vi "Periodic Tasks.vi"(8 "error in":errorcluster) -> ()   [LabVIEW 2016]
doc: "This VI runs in parallel to other tasks. It can contain as many user-defined periodic loops as you need. These can carry out PID or other sorts of timed response."
uses:
  Common Code/Goal Vision Packet.ctl
  Common Code/Utilities/TimeManager.vi
  Common Code/Utilities/Change Detect.vi
  Common Code/Utilities/Change Detect Boolean.vi
  Robot Global Data.vi
  <vilib>/Rock Robotics/WPI/Utilities/WPI_GetSetVariantRefNum.vi
panel:
  # "e"
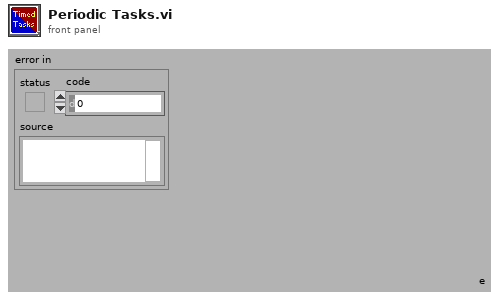
[diagram p1: front panel]
types:
  T1 = typedef "WPI_DriverStationRobotMode2.ctl" = enum16{"Autonomous Disabled", "Autonomous Enabled", "Teleop Disabled", "Teleop Enabled", "Disconnected", "Finish", "Test Disabled", "Test Enabled", "Emergency Stopped"}
  T2 = typedef "WPI_JoystickDevRef.ctl" = cluster{"Device":T3}
  T3 = typedef "WPI_JoystickDeviceEnum.ctl" = enum16{"USB 0", "USB 1", "USB 2", "USB 3", "USB 4", "USB 5"}
  T4 = typedef "D-Pad.ctl" = cluster{"Top":bool, "Bottom":bool, "None":bool, "Right":bool, "Left":bool}
  T5 = typedef "Button Cluster.ctl" = cluster{"Buttons[0]":bool, "Buttons[1]":bool, "Buttons[2]":bool, "Buttons[3]":bool, "Buttons[4]":bool, "Buttons[5]":bool, "Buttons[6]":bool, "Buttons[7]":bool, "Buttons[8]":bool, "Buttons[9]":bool}
  T6 = typedef "Goal Vision Packet.ctl" = cluster{"Distance":dbl, "Angle":dbl, "Found Target?":bool}
  T7 = typedef "Dashboard Control Data.ctl" = cluster{"Drivetrain Settings":T8, "Intake Presets ":T10, "Shooter Presets":T11, "Vision Target Packet":T12, "Auton Presets":cluster{"Start Position":dbl}, "Drivetrain Encoder Values":T13, "Drivetrain Encoder Settings":cluster{"Left Tick Constant":dbl, "Right Tick Contant":dbl, "Reset Encoders":bool, "Center Tick Constant":dbl}, "Zero Gyro":bool, "Vision Timeout":dbl}
  T8 = typedef "Drivetrain Settings.ctl" = cluster{"Gyro Tolerance":dbl, "Gyro Steer PID Gains":T9, "Y Power Multiplier":dbl, "Turn Power Multiplier":dbl, "Gyro Output":dbl, "Creep Rate":dbl, "Distance Drive PID Gains":T9, "Distance Tolerance":dbl, "Distance Output":dbl, "Strafe Threshold":dbl, "Strafe Correct":bool, "Strafe Corect Tolerance":dbl, "Translate Drive PID Gains":T9, "Strafe Output":dbl, "SC Right":dbl, "SC Left":dbl, "Use Gyro":bool, "Constant Power":bool, "Strafe Power":dbl}
  T9 = typedef "PID Gains.ctl" = cluster{"proportional gain (Kc)":dbl, "integral time (Ti, min)":dbl, "derivative time (Td, min)":dbl}
  T10 = typedef "Intake Presets.ctl" = cluster{"Intake Speed ":dbl, "Outake Speed":dbl, "Current Trip Delay":dbl, "Max Current":dbl}
  T11 = typedef "Shooter Presets.ctl" = cluster{"Key Shot":cluster{"RPM ":dbl, "Hood?":bool}, "Distance Shot":cluster{"RPM":dbl, "Hood?":bool}, "RPM Tolerance":dbl, "Unstuck Delay Time ":dbl, "Initial RPM Increase":dbl, "Warmup Delay":dbl, "Faster Time":dbl, "Shooter PID Gains":cluster{"P":dbl, "I":dbl, "D":dbl, "FF":dbl, "Ramp Rate":dbl, "I Zone":dbl}}
  T12 = typedef "Vision Target Packet.ctl" = cluster{"Robot Center":dbl, "Center X":dbl, "Center Y":dbl, "Angle":dbl, "Distance":dbl, "Found Target?":bool}
  T13 = typedef "Drivetrain Encoder Values.ctl" = cluster{"Left Encoder":T14, "Center Encoder":T14, "Right Encoder":T14}
  T14 = typedef "Encoder Values.ctl" = cluster{"Distance":dbl, "Speed":dbl, "Tick":dbl}
  T15 = typedef "WPI_CameraDevRef.ctl" = cluster{"Camera Address":string, "CameraStatus":errorcluster}
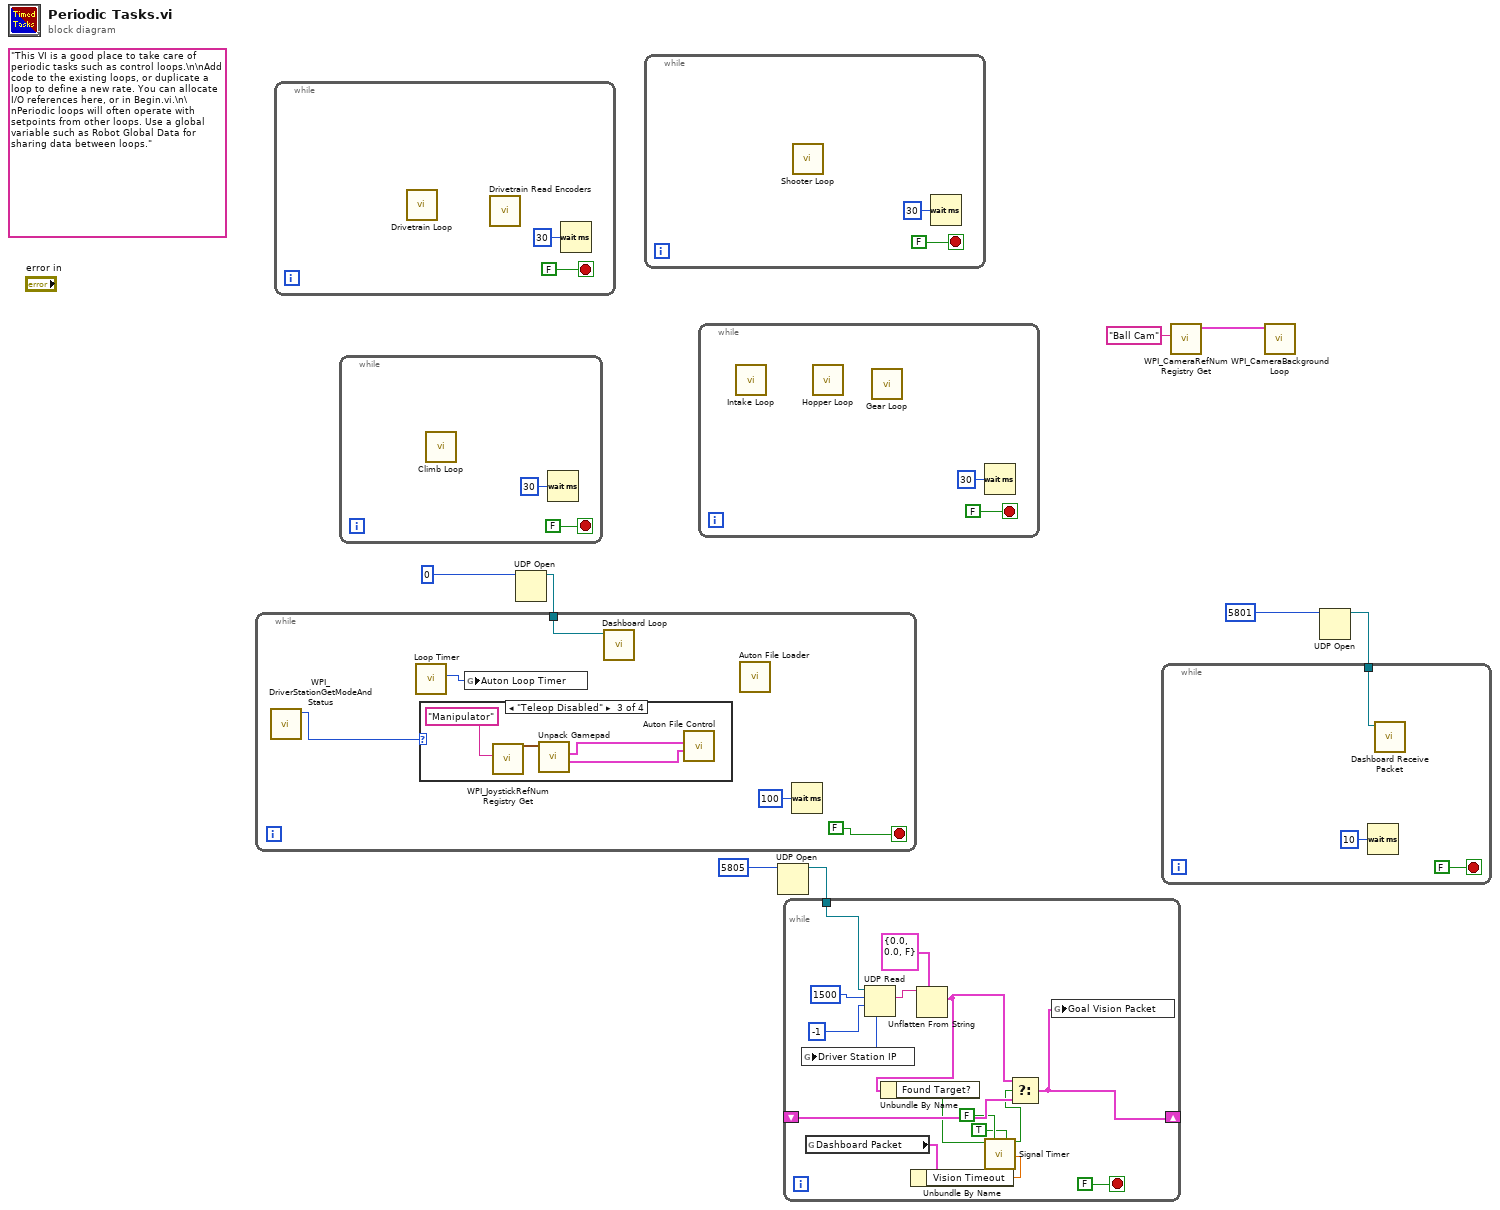
[diagram p0: block diagram]
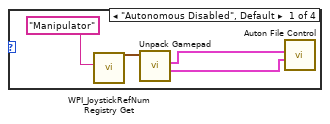
[diagram p2: hidden frame]
diagram:
  (unwired) "This VI is a good place to take care of periodic tasks such as control loops.\n\nAdd code to the existing loops, or duplicate a loop to define a new rate. You can allocate I/O references here, or in Begin.vi.\n\nPeriodic loops will often operate with setpoints from other loops. Use a global variable such as Robot Global Data for sharing data between loops."
  n1 = while {
    stop <- FALSE stop-if-true
    n2 = call "Drivetrain Loop.vi"() -> ()  [unwired: 12 in]
    n3 = call "Drivetrain Read Encoders.vi"() -> ()  [unwired: 11 in, 1 out]
    n4 = Wait (ms)(milliseconds to wait=u32 30) -> ()  [unwired: 1 out]
  }
  n5 = while {
    stop <- FALSE stop-if-true
    n6 = call "Climb Loop.vi"() -> ()  [unwired: 12 in]
    n7 = Wait (ms)(milliseconds to wait=u32 30) -> ()  [unwired: 1 out]
  }
  n8 = UDP Open(11:0) -> (port=w6:refnum<k16>)  [unwired: 4 in, 2 out]
  n9 = while {
    tunnel: w6 -> [w15]
    stop <- FALSE stop-if-true
    n10 = call <vilib>:"WPI_DriverStationGetModeAndStatus.vi"() -> ("Robot Mode"=w13:T1)  [unwired: 10 in, 1 out]
    n11 = call "Loop Timer.vi"() -> ("dt"=w14:u32)  [unwired: 11 in]
    n12 = case shown="\"Teleop Disabled\"" w13 {
      frame "Autonomous Disabled", Default {
        n13 = call <vilib>:"WPI_JoystickRefNum Registry Get.vi"("refnum name"="Manipulator") -> ("JoystickDevRef"=w20:T2)  [unwired: 9 in, 1 out]
        n14 = call "Unpack Gamepad.vi"("JoystickDevRef"=w20) -> ("D-Pad"=w18:T4, "Button Cluster"=w19:T5)  [unwired: 8 in, 1 out]
        n15 = call "Auton File Control.vi"("D-Pad"=w18, "Button Cluster"=w19) -> ()  [unwired: 10 in]
      }
      frame "Autonomous Enabled" {
        # "nothing :)"
      }
      frame "Teleop Disabled" {
        n16 = call <vilib>:"WPI_JoystickRefNum Registry Get.vi"("refnum name"="Manipulator") -> ("JoystickDevRef"=w24:T2)  [unwired: 9 in, 1 out]
        n17 = call "Unpack Gamepad.vi"("JoystickDevRef"=w24) -> ("D-Pad"=w22:T4, "Button Cluster"=w23:T5)  [unwired: 8 in, 1 out]
        n18 = call "Auton File Control.vi"("D-Pad"=w22, "Button Cluster"=w23) -> ()  [unwired: 10 in]
      }
      frame "Teleop Enabled" {
      }
    }
    n19 = global write "Robot Global Data.vi" "Auton Loop Timer"(w14) -> ()
    n20 = call "Dashboard Loop.vi"("connection ID"=w15) -> ()  [unwired: 11 in]
    n21 = call "Auton File Loader.vi"() -> ()  [unwired: 12 in]
    n22 = Wait (ms)(milliseconds to wait=u32 100) -> ()  [unwired: 1 out]
  }
  n23 = while {
    stop <- FALSE stop-if-true
    n24 = call "Shooter Loop.vi"() -> ()  [unwired: 12 in]
    n25 = Wait (ms)(milliseconds to wait=u32 30) -> ()  [unwired: 1 out]
  }
  n26 = while {
    stop <- FALSE stop-if-true
    n27 = call "Intake Loop.vi"() -> ()  [unwired: 12 in]
    n28 = call "Hopper Loop.vi"() -> ()  [unwired: 12 in]
    n29 = call "Gear Loop.vi"() -> ()  [unwired: 12 in]
    n30 = Wait (ms)(milliseconds to wait=u32 30) -> ()  [unwired: 1 out]
  }
  n31 = UDP Open(11:5805) -> (port=w3:refnum<k16>)  [unwired: 4 in, 2 out]
  n32 = while {
    tunnel: w3 -> [w45]
    shift-right: [w37] -> _
    shift-left: _ -> [w38]
    stop <- FALSE stop-if-true
    n33 = global read "Robot Global Data.vi" "Dashboard Packet"() -> (w31:T7)
    n34 = UDP Read(connection ID=w45, max size (548)=1500, timeout ms (25000)=-1) -> (data out=w41:string, 6:w42:u32)  [unwired: 1 in, 3 out]
    n35 = global write "Robot Global Data.vi" "Driver Station IP"(w42) -> ()
    n36 = Unbundle By Name(w31) -> ("Vision Timeout"=w30:dbl)
    n37 = Unflatten From String(type=T6 {"Distance"=0.0, "Angle"=0.0, "Found Target?"=FALSE} ("Goal Vision Packet"), binary string=w41) -> (value=w36:T6)  [unwired: 3 in, 2 out]
    n38 = Unbundle By Name(w36) -> ("Found Target?"=w35:bool)
    n39 = call "Signal Timer.vi"("Input"=w35, "Edge"=FALSE, "Interval"=w30, "Pull"=TRUE) -> ("Filtered Output"=w32:bool)  [unwired: 11 in]
    n40 = Select(t=w36, s=w32, f=w38) -> (s? t:f=w37:T6)
    n41 = global write "Robot Global Data.vi" "Goal Vision Packet"(w37) -> ()
  }
  n42 = call <vilib>:"WPI_CameraRefNum Registry Get.vi"("refnum name"="Ball Cam") -> ("CameraDevRef"=w2:T15)  [unwired: 9 in, 1 out]
  n43 = call <vilib>:"WPI_CameraBackground Loop.vi"("CameraDevRef"=w2) -> ()  [unwired: 11 in]
  n44 = UDP Open(11:5801) -> (port=w5:refnum<k16>)  [unwired: 4 in, 2 out]
  n45 = while {
    tunnel: w5 -> [w47]
    stop <- FALSE stop-if-true
    n46 = Wait (ms)(milliseconds to wait=u32 10) -> ()  [unwired: 1 out]
    n47 = call "Dashboard Receive Packet.vi"("connection ID"=w47) -> ()  [unwired: 11 in]
  }
